vi "Create_Device.vi"(8 "error in (no error)":errorcluster, 9 "Number of Slots":i8, 10 "Device Name":string) -> (0 "error out":errorcluster, 3 "87Pn out":refnum<class "USB-87Pn.lvclass">)   [LabVIEW 2019, in "USB-87Pn.lvlib" / "USB-87Pn.lvclass"]
doc: "The purpose of this section to to create a new 87Pn device for configuration."
uses:
  USB-87Pn.lvclass
  Module/AI_Module_Data.ctl
  Module/Module_Data.ctl
  Module/DO_Module_Data.ctl
  USB-87Pn.lvclass/USB-87Pn.ctl
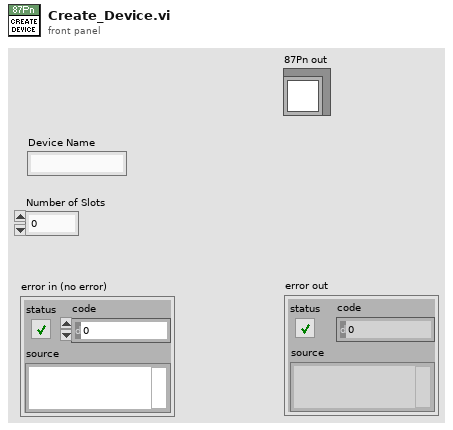
[diagram p1: front panel]
types:
  T1 = typedef "USB-87Pn.lvlib/USB-87Pn.lvclass/DO_Module_Data.ctl" = cluster{"Module_Data":T2, "DO_Channels":cluster{"Enabled":bool, "Alias":string}[]}
  T2 = typedef "USB-87Pn.lvlib/USB-87Pn.lvclass/Module_Data.ctl" = cluster{"Number of Channels":u8, "Address":i16, "Alias":string}
  T3 = typedef "USB-87Pn.lvlib/USB-87Pn.lvclass/AI_Module_Data.ctl" = cluster{"Module_Data":T2, "AI_Channels":cluster{"Enabled":bool, "Alias":string}[]}
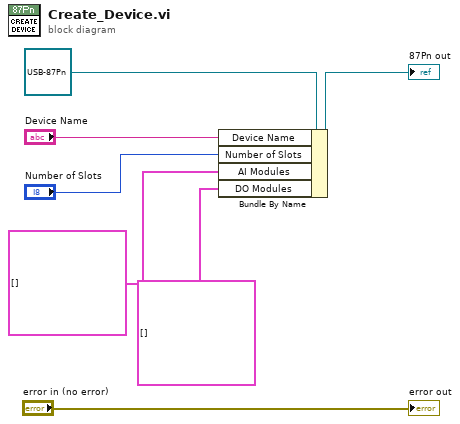
[diagram p0: block diagram]
diagram:
  n1 = Bundle By Name(cluster=refnum<class "USB-87Pn.lvclass"> refnum ("USB-87Pn.lvlib:USB-87Pn.lvclass"), "Device Name"="Device Name", "Number of Slots"="Number of Slots", "AI Modules"=T3[] [], "DO Modules"=T1[] []) -> (→"87Pn out":refnum<class "USB-87Pn.lvclass">)
  "error out" <- "error in (no error)"
